vi "Dashboard Main.vi"() -> ()   [LabVIEW 2015]
uses:
  <vilib>/Utility/miscctls.llb/LVRowAndColumnTypeDef.ctl
  <vilib>/event_ctls.llb/eventvkey.ctl
  <vilib>/Rock Robotics/WPI/Dashboard/WPI_DashboardLogging Global.vi
  <vilib>/Rock Robotics/Network Tables/NT Read Numeric Array.vi
  <vilib>/Rock Robotics/Network Tables/NT Write Boolean.vi
  <vilib>/Utility/config.llb/Write Key (String).vi
  <vilib>/Utility/config.llb/Write Key (I32).vi
  <vilib>/Utility/config.llb/NI_LVConfig.lvlib
panel:
  in  "TCP":refnum<k5>
  in  "Rec Mode":enum32{"Stop", "Record", "Playback"}(radio)
  in  "Vision":u16(ring) items=["Camera Off", "USB Camera SW", "USB Camera HW", "IP Camera"]
  out "Camera IP":string
  out "Image Message":string="Timeout in Camera Communications"
  in  "Dashboard Tab":T1(tab)
  in  "Select Auto":string(combo)
  out "NT Connection":bool
  in  "Camera Settings":T2={"Frame Rate"=30, "Compression"=30, "Size"=1} {"Frame Rate" scale=1.0..30.0; "Size" items=["640x480", "320x240", "160x120"]}
  out "MotorChart R":cluster{"Numeric":dbl, "Numeric":dbl}(graph)
  out "MotorChart L":T3(graph)
  out "MotorSliders R":cluster{"MotorSlide1":dbl, "MotorSlide2":dbl} {"MotorSlide2" scale=-1.0..1.0 scale format="%#_2e"; "MotorSlide1" scale=-1.0..1.0 scale format="%#_2e"}
  out "MotorSliders L":T4 {"MotorSlide4 2" scale=0.0..14.0 scale format="%#_2e"; "MotorSlide2" scale=-1.0..1.0 scale format="%#_2e"; "MotorSlide1" scale=-1.0..1.0 scale format="%#_2e"}
  out "Gyro":dbl(knob) scale=0.0..360.0
  out "JS1 Z":dbl(slide) scale=-1.0..1.0 scale format="%#_2e"
  out "JS1 Graph":cluster{"X":dbl, "Y":dbl}[](graph)
  out "JS1 Buttons":T5
  out "JS2 Z":dbl(slide) scale=-1.0..1.0 scale format="%#_2e"
  out "JS2 Graph":cluster{"X":dbl, "Y":dbl}[](graph)
  out "JS2 Buttons":T5
  out "Mode":T6(ring)=enum."Auto Disabled"
  in  "DB Camera Config":bool
  out "fps":dbl format="%#.1g"
  out "Mbps":dbl format="%#.1g"
  out "Mbps LED":bool
  in  "Camera Switch":bool
  in  "Defenses":T7(ring)
  in  "Position":T8(ring)
  in  "DB/String 9":string
  in  "DB/String 8":string
  in  "DB/String 7":string
  in  "DB/String 6":string
  in  "DB/String 5":string
  in  "DB/String 4":string
  in  "DB/String 3":string
  in  "DB/String 2":string
  in  "DB/String 1":string
  in  "DB/String 0":string
  in  "DB/Slider 0":dbl(slide) scale=0.0..5.0
  in  "DB/Slider 1":dbl(slide) scale=0.0..5.0
  in  "DB/Slider 2":dbl(slide) scale=0.0..5.0
  in  "DB/Slider 3":dbl(slide) scale=0.0..5.0
  out "DB/LED 3":bool
  out "DB/LED 2":bool
  out "DB/LED 1":bool
  out "DB/LED 0":bool
  in  "DB/Button 3":bool
  in  "DB/Button 2":bool
  in  "DB/Button 1":bool
  in  "DB/Button 0":bool caption="New Name"
  in  "Test Slider":dbl(slide) scale=0.0..100.0 scale format="%#_3g"
  in  "On/Off":bool caption="Solenoid"
  in  "Test Name":u16(ring) items=["Select the test to run..."]
  in  "Test Tree":string(tree)
  in  "Motor":cluster{"Value":dbl, "Enable":bool} {"Value" scale=-1.0..1.0 scale format="%#_3g"}
  out "Progress":T9 {"Test Progress" scale=0.0..100.0}
  in  "Rev/Fwd":cluster{"Forward":bool, "Reverse":bool}
  in  "Test Ring":u16(ring) items=["Monochrome", "Color"]
  out "Cmd Status":string
  in  "Execute Command":bool
  in  "Command Params":string[][](table)
  in  "Command Selection":i32(listbox)
  in  "CheckList":i32(listbox)
  out "Tree":string(tree)
  out "Camera Image":T10(plugin-control)
  # "Left"
  # "Front"
  # "Right"
  # "Battery"
  # "This tab is a great place for autonomous settings and robot-specific values.\nPlace controls and indicators inside this tab and match name to\nDashboard Variables on robot. You can also delete this comment."
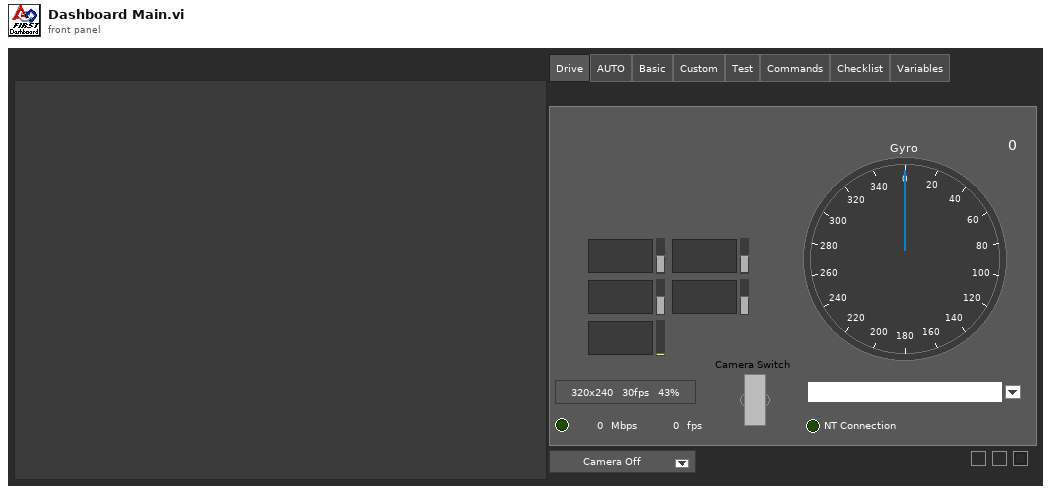
[diagram p1: front panel]
types:
  T1 = enum32{"Drive", "AUTO", "Basic", "Custom", "Test", "Commands", "Checklist", "Variables"}
  T2 = cluster{"Frame Rate":i32, "Compression":i32, "Size":u16}
  T3 = cluster{"Numeric":dbl, "Numeric":dbl, "Battery V":dbl}
  T4 = cluster{"MotorSlide1":dbl, "MotorSlide2":dbl, "MotorSlide4 2":dbl}
  T5 = cluster{bool, bool, bool, bool, bool, bool, bool, bool, bool, bool, bool, bool}
  T6 = enum8{"Tele-Op Disabled", "Tele-Op Enabled", "Auto Disabled", "Auto Enabled", "Test Disabled", "Test Enabled", "Disconnected", "No Code", "E-Stop"}
  T7 = enum16{"Sally Port", "Portcullis", "Drawbridge", "Moat", "Rock Wall", "Cheval De Frise", "Ramparts", "Low Bar", "Rocky Terrain"}
  T8 = enum16{"Position 5", "Position 4", "Position 3", "Position 2", "Position 1"}
  T9 = cluster{"Test Progress":u8, "Test Progress Text":string}
  T10 = typedef "IMAQ Image.ctl" = refnum<image>
  T11 = cluster{"IDs":cluster{"RPC field ID":u16, "Unique ID":u16}, "String":string}
  T12 = enum32{"Drive", "Basic", "Custom", "Test", "Checklist", "Variables"}
  T13 = typedef "Image Type" = u32
  T14 = cluster{"Error Strings":string, "Disable Counts":cluster{u16, u16}, "Rail Faults":cluster{u16, u16, u16}, "Robot IP":string, "DB Mode":u8, "Event Info":cluster{"Name":string, "Type":u8, "Number":u16, "Replay":u8}, "Camera Addr":string}
  T15 = cluster{"Storage":cluster{"Disk Free":u64, "RAM Block":u32, "RAM free":u32}, "CPU Utilization":cluster{"CPU % ISR":sgl, "CPU % Time Crit":sgl, "CPU % Timed Str":sgl, "CPU % High":sgl, "CPU % Above":sgl, "CPU % Normal":sgl, "CPU % Low":sgl}, "CAN":cluster{"% Bus Utilization":sgl, "Bus Off Cnt":u32, "TX_FIFO Full Cnt":u32, "Receive Error Cnt":u8, "Transmit Error Cnt":u8}, "HID":cluster{"HID Outputs":u32, "Rumble Low":u16, "Rumble High":u16}[]}
  T16 = cluster{"Status bits":cluster{"Test Mode":bool, "Autonomous":bool, "Enabled":bool, "Code Start":bool, "Brownout":bool, "Reserved 2":bool, "Reserved 3":bool, "E-Stop":bool}, "Code Trace":cluster{"Disabled":bool, "TeleOp":bool, "Auto":bool, "Test":bool}, "Controller Type":enum16{"unknown", "cRIO", "roboRio"}, "Code?":enum16{"unknown", "noCode", "code"}, "Battery V":dbl}
  T17 = cluster{"Control Bits":cluster{"TestMode":bool, "Autonomous":bool, "Enabled":bool, "FMS Present":bool, bool, bool, bool, "E-Stop":bool}, "Team Station ":u8, "Countdown":sgl, "Joystick Values":cluster{"Axes":dbl[], "Buttons":bool[], "POVs":i16[]}[]}
  T18 = cluster{"Axes":dbl[], "Buttons":bool[], "POVs":i16[]}[]
  T19 = cluster{"Axes":dbl[], "Buttons":bool[], "POVs":i16[]}
  T20 = cluster{"Buttons[0]":bool, "Buttons[1]":bool, "Buttons[2]":bool, "Buttons[3]":bool, "Buttons[4]":bool, "Buttons[5]":bool, "Buttons[6]":bool, "Buttons[7]":bool, "Buttons[8]":bool, "Buttons[9]":bool, "Buttons[10]":bool, "Buttons[11]":bool}
  T21 = typedef "NI_LVConfig.lvlib/Config Data RefNum.ctl" = refnum<k1>
  T22 = cluster{"Operation":enum16{"Update", "Clear"}, "Color Box":u32}[]
  T23 = typedef "eventvkey.ctl" = enum16{"ASCII", "Enter", "Return", "Shift", "Ctrl", "Alt", "Cmd", "Opt", "Caps", "NumLock", "Clear", "Break", "Up", "Down", "Left", "Right", "Insert", "Delete", "Home", "End", "PageUp", "PageDown", "Escape", "Help", "Pause", "ScrollLock", "F1", "F2", "F3", "F4", "F5", "F6", "F7", "F8", "F9", "F10", "F11", "F12", "F13", "F14", "F15", "F16", "F17", "F18", "F19", "F20", "F21", "F22", "F23", "F24", "Play", "VolumeUp", "VolumeDown", "Mute", "Two Byte Char"}
  T24 = cluster{"Image Size":bool, "Image Type":bool, "Pixel Value":bool, "ROI Information":bool, "Zoom Factor":bool}
  T25 = enum8{"Enabled", "Disabled", "Disabled and Grayed Out"}
  T26 = cluster{"Operation":enum16{"Update", "Clear"}, "Color Box":u32}
  T27 = typedef "LVRowAndColumnTypeDef.ctl" = cluster{"Row":i32, "Column":i32}
  T28 = cluster{"Shift":bool, "Ctrl":bool, "Alt":bool, "Cmd":bool, "Opt":bool}
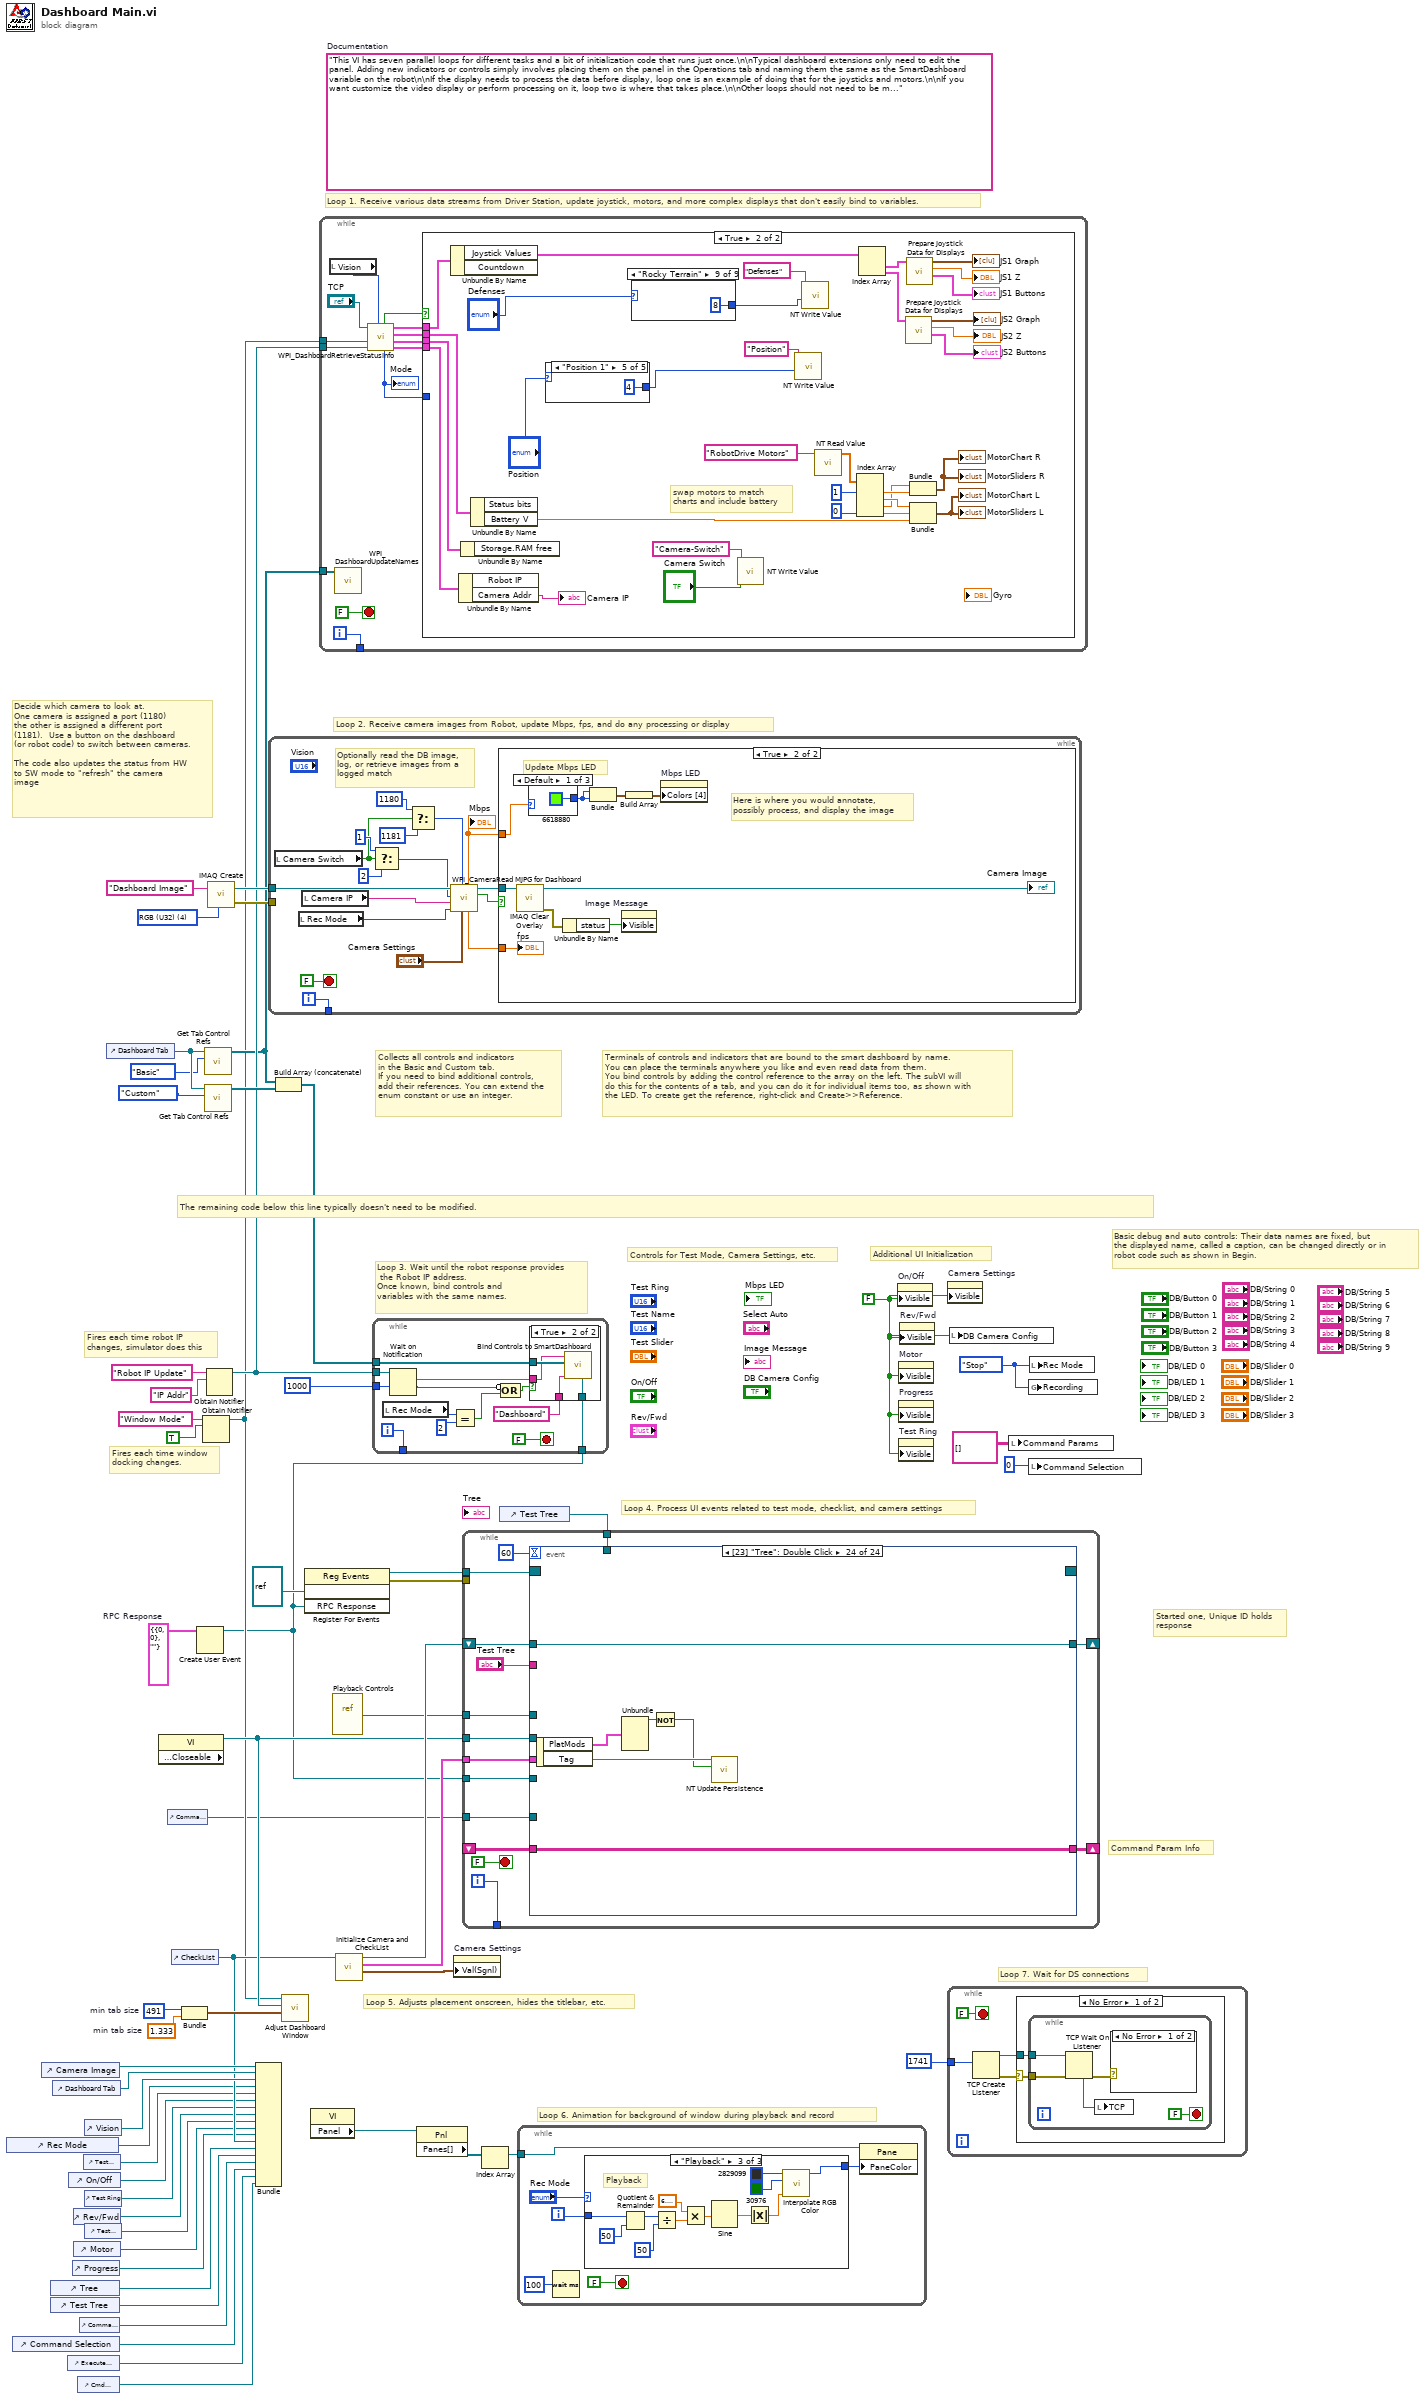
[diagram p0: block diagram]
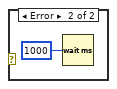
[diagram p2: hidden frame]
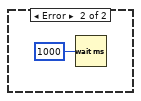
[diagram p3: hidden frame]
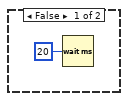
[diagram p4: hidden frame]
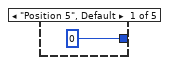
[diagram p5: hidden frame]
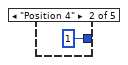
[diagram p6: hidden frame]
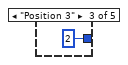
[diagram p7: hidden frame]
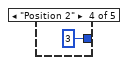
[diagram p8: hidden frame]
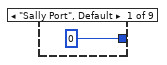
[diagram p9: hidden frame]
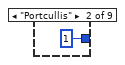
[diagram p10: hidden frame]
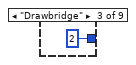
[diagram p11: hidden frame]
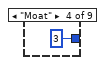
[diagram p12: hidden frame]
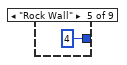
[diagram p13: hidden frame]
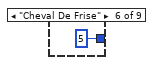
[diagram p14: hidden frame]
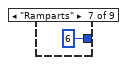
[diagram p15: hidden frame]
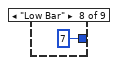
[diagram p16: hidden frame]
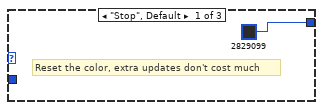
[diagram p17: hidden frame]
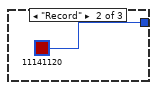
[diagram p18: hidden frame]
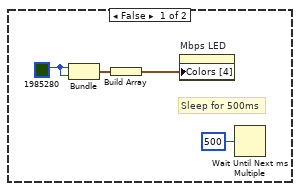
[diagram p20: hidden frame]
diagram:
  w7 = T11 {"IDs"={"RPC field ID"=0, "Unique ID"=0}, "String"=""}  # RPC Response
  w30 = 491  # min tab size
  w29 = 1.333  # min tab size
  w38 = enum32{"Stop", "Record", "Playback"}."Stop" ("Rec Mode")
  w14 = FALSE ("Visible")
  (unwired) "This VI has seven parallel loops for different tasks and a bit of initialization code that runs just once.\n\nTypical dashboard extensions only need to edit the panel. Adding new indicators or controls simply involves placing them on the panel in the Operations tab and naming them the same as the SmartDashboard variable on the robot\n\nIf the display needs to process the data before display, loop one is an example of doing that for the joysticks and motors.\n\nIf you want customize the video display or perform processing on it, loop two is where that takes place.\n\nOther loops should not need to be modified. They are pretty standard, and document the task they perform."  # Documentation
  w58 = T13 4 items=["Grayscale (U8)", "Grayscale (I16)", "Grayscale (SGL)", "Complex (CSG)", "RGB (U32)", "HSL (U32)", "RGB (U64)"] ("Image Type")
  # "Decide which camera to look at.\nOne camera is assigned a port (1180)\nthe other is assigned a different port\n(1181).  Use a button on the dashboard\n(or robot code) to switch between cameras.\n\nThe code also updates the status from HW\nto SW mode to \"refresh\" the camera\nimage"
  # "Command Param Info"
  # "Started one, Unique ID holds\nresponse"
  # "Loop 7. Wait for DS connections"
  # "Basic debug and auto controls: Their data names are fixed, but\nthe displayed name, called a caption, can be changed directly or in\nrobot code such as shown in Begin."
  # "Controls for Test Mode, Camera Settings, etc."
  # "Additional UI Initialization"
  # "Loop 6. Animation for background of window during playback and record"
  # "Fires each time robot IP\nchanges, simulator does this"
  # "Fires each time window\ndocking changes."
  # "Collects all controls and indicators\nin the Basic and Custom tab.\nIf you need to bind additional controls,\nadd their references. You can extend the\nenum constant or use an integer."
  # "The remaining code below this line typically doesn't need to be modified."
  # "Loop 4. Process UI events related to test mode, checklist, and camera settings"
  # "Terminals of controls and indicators that are bound to the smart dashboard by name.\nYou can place the terminals anywhere you like and even read data from them.\nYou bind controls by adding the control reference to the array on the left. The subVI will\ndo this for the contents of a tab, and you can do it for individual items too, as shown with\nthe LED. To create get the reference, right-click and Create>>Reference."
  # "Loop 3. Wait until the robot response provides\n the Robot IP address.\nOnce known, bind controls and\nvariables with the same names."
  # "Loop 5. Adjusts placement onscreen, hides the titlebar, etc."
  # "Loop 1. Receive various data streams from Driver Station, update joystick, motors, and more complex displays that don't easily bind to variables."
  # "Loop 2. Receive camera images from Robot, update Mbps, fps, and do any processing or display"
  n1 = control-ref of="Rec Mode"() -> (w20:refnum<vi>)
  n2 = control-ref of="Command Selection"() -> (w6:refnum<vi>)
  n3 = control-ref of="Camera Image"() -> (w33:refnum<vi>)
  n4 = control-ref of="Tree"() -> (w24:refnum<vi>)
  n5 = control-ref of="Test Tree"() -> (w23:refnum<vi>)
  n6 = control-ref of="Dashboard Tab"() -> (w32:refnum<vi>)
  n7 = control-ref of="Execute Command"() -> (w8:refnum<vi>)
  n8 = control-ref of="On/Off"() -> (w18:refnum<vi>)
  n9 = control-ref of="Progress"() -> (w15:refnum<vi>)
  n10 = control-ref of="Rev/Fwd"() -> (w16:refnum<vi>)
  n11 = control-ref of="Motor"() -> (w21:refnum<vi>)
  n12 = control-ref of="Cmd Status"() -> (w2:refnum<vi>)
  n13 = control-ref of="Command Params"() -> (w9:refnum<vi>)
  n14 = control-ref of="Test Slider"() -> (w19:refnum<vi>)
  n15 = control-ref of="Vision"() -> (w31:refnum<vi>)
  n16 = control-ref of="Test Ring"() -> (w17:refnum<vi>)
  n17 = control-ref of="Test Name"() -> (w22:refnum<vi>)
  n18 = control-ref of="Dashboard Tab"() -> (w36:refnum<vi>)
  n19 = property class="VI" props=["Front Panel.Closeable"]() -> (reference out=w37:refnum<vi>)  [unwired: 2 in, 2 out]
  n20 = control-ref of="Command Params"() -> (w1:refnum<vi>)
  n21 = control-ref of="CheckList"() -> (w25:refnum<vi>)
  n22 = Bundle("min tab size"=w30, "min tab size"=w29) -> (w28:cluster{"min tab size":i32, "min tab size":dbl})  [unwired: 1 in]
  n23 = Create User Event(user event datatype=w7) -> (user event=w3:refnum<user-event>)  [unwired: 1 in, 1 out]
  n24 = Obtain Notifier(name (unnamed)="Window Mode", notification data type=TRUE) -> (notifier out=w11:refnum<notifier>)  [unwired: 2 in, 2 out]
  n25 = call <vilib>:"Get Tab Control Refs.vi"("Page Index"=T12."Basic" ("Dashboard Tab"), "TabControl in"=w36) -> ("ControlsOnPage"=w12:refnum<vi>[])  [unwired: 9 in]
  n26 = call <vilib>:"Get Tab Control Refs.vi"("Page Index"=T12."Custom" ("Dashboard Tab"), "TabControl in"=w36) -> ("ControlsOnPage"=w35:refnum<vi>[])  [unwired: 9 in]
  n27 = Obtain Notifier(name (unnamed)="Robot IP Update", notification data type="IP Addr" ("name (unnamed)")) -> (notifier out=w13:refnum<notifier>)  [unwired: 2 in, 2 out]
  n28 = call "IMAQ Create"("Image Name"="Dashboard Image", "Image Type"=w58) -> ("New Image"=w56:T10, "error out"=w55:errorcluster)  [unwired: 2 in, 1 out]
  n29 = Bundle("Camera Image"=w33, "Dashboard Tab"=w32, "Vision"=w31, "Rec Mode"=w20, "Test Slider"=w19, "On/Off"=w18, "Test Ring"=w17, "Rev/Fwd"=w16, "Test Name"=w22, "Motor"=w21, "Progress"=w15, "CheckList"=w25, "Tree"=w24, "Test Tree"=w23, "Command Params"=w9, "Command Selection"=w6, "Execute Command"=w8, "Cmd Status"=w2) -> ()  [unwired: 1 in, 1 out]
  n30 = while {
    tunnel: w56 -> [w73]
    tunnel: w55 -> [_]
    tunnel: [w74] -> _
    i -> [w74]
    stop <- FALSE stop-if-true
    # "Optionally read the DB image,\nlog, or retrieve images from a\nlogged match"
    n31 = local read "Camera Switch"() -> (w60:bool)
    n32 = local read "Rec Mode"() -> (w68:enum32{"Stop", "Record", "Playback"})
    n33 = local read "Camera IP"() -> (w67:string)
    n34 = Select(t=1, s=w60, f=2) -> (s? t:f=w63:i32)
    n35 = Select(t=1180, s=w60, f=1181) -> (s? t:f=w59:i32)
    n36 = call <vilib>:"WPI_CameraRead MJPG for Dashboard.vi"("Camera Settings"="Camera Settings", "Camera Port"=w59, "Rec Mode"=w68, "Camera IP"=w67, "Camera Mode"=w63, "Refnum in"=w73) -> ("Active"=w71:bool, "Refnum out"=w72:T10, "FPS"=w70:dbl, "Bandwidth (Mbps)"=w66:dbl)  [unwired: 2 in]
    "Mbps" <- w66
    n37 = case shown="True" w71 {
      tunnel: w72 -> [_ w83]
      tunnel: w66 -> [_ w82]
      tunnel: w70 -> [_ w80]
      frame False {
        w76 = u32 1985280 ("Color Box")
        # "Sleep for 500ms"
        n38 = Bundle("Color Box"=w76, "Color Box"=w76) -> (w78:cluster{"Color Box":u32, "Color Box":u32})  [unwired: 1 out]
        n39 = Build Array(w78) -> (w77:cluster{"Color Box":u32, "Color Box":u32}[])
        n40 = property on="Mbps LED" class="Bool (strict)"("Colors [4]"=w77) -> ()  [unwired: 2 in, 2 out]
        n41 = Wait Until Next ms Multiple(millisecond multiple=u32 500) -> ()  [unwired: 1 out]
      }
      frame True {
        # "Here is where you would annotate,\npossibly process, and display the image"
        # "Update Mbps LED"
        n42 = call "IMAQ Clear Overlay"("Image"=w83) -> ("error out"=w87:errorcluster, "Image Out"=→"Camera Image":T10)  [unwired: 2 in, 7 out]
        n43 = case shown="Default" w82 {
          tunnel: [u32 6618880 ("Color Box") u32 16776722 ("Color Box") u32 16716800 ("Color Box")] -> w84
          frame Default {
          }
          frame 4, 5 {
          }
          frame 6.. {
          }
        }
        n44 = Unbundle By Name(w87) -> ("status"=w88:bool)
        n45 = Bundle("Color Box"=w84, "Color Box"=w84) -> (w86:cluster{"Color Box":u32, "Color Box":u32})  [unwired: 1 out]
        n46 = property on="Image Message" class="Str"("Visible"=w88) -> ()  [unwired: 2 in, 2 out]
        n47 = Build Array(w86) -> (w85:cluster{"Color Box":u32, "Color Box":u32}[])
        n48 = property on="Mbps LED" class="Bool (strict)"("Colors [4]"=w85) -> ()  [unwired: 2 in, 2 out]
        "fps" <- w80
      }
    }
  }
  n49 = Build Array (concatenate)(w12, w35) -> (w34:refnum<vi>[])
  n50 = call "Adjust Dashboard Window.vi"("Size Constraints"=w28, "VI"=w37, "WIn Mode"=w11) -> ()  [unwired: 9 in]
  n51 = register-events(refnum<vi> refnum, w3) -> (reference out=w42:refnum<event-registration>, error out=w41:errorcluster)  [unwired: 2 in]
  n52 = property class="VI"() -> ("Panel"=w45:refnum<vi>)  [unwired: 2 in, 2 out]
  n53 = while {
    tunnel: [w103] -> _
    tunnel: w13 -> [w97]
    tunnel: w12 -> [w96]
    tunnel: w11 -> [w92]
    i -> [w103]
    stop <- FALSE stop-if-true
    n54 = local read "Vision"() -> (w94:u16)
    n55 = call <vilib>:"WPI_DashboardUpdateNames.vi"("Controls on Tab"=w96) -> ()  [unwired: 11 in]
    n56 = call <vilib>:"WPI_DashboardRetrieveStatusInfo.vi"("Vision"=w94, "Binding Refnum"=w97, "Window Mode Notifier"=w92, "TCP Cnx"="TCP") -> ("Power and Errors"=w98:T14, "Robot Metrics"=w101:T15, "Status Info"=w102:T16, "Control Info"=w99:T17, "Robot Mode"=w95:T6, "Process?"=w100:bool)  [unwired: 2 in]
    "Mode" <- w95
    n57 = case shown="True" w100 {
      tunnel: w102 -> [_ w138]
      tunnel: w101 -> [_ w137]
      tunnel: w99 -> [_ w136]
      tunnel: w98 -> [_ w135]
      tunnel: w95 -> [_ _]
      frame False {
        n58 = Wait (ms)(milliseconds to wait=u32 20) -> ()  [unwired: 1 out]
      }
      frame True {
        # "swap motors to match\ncharts and include battery"
        n59 = Unbundle By Name(w136) -> ("Joystick Values"=w125:T18)  [unwired: 1 out]
        n60 = Unbundle By Name(w135) -> ("Camera Addr"=→"Camera IP":string)  [unwired: 1 out]
        n61 = Unbundle By Name(w137) -> ()  [unwired: 1 out]
        n62 = Unbundle By Name(w138) -> ("Battery V"=w126:dbl)  [unwired: 1 out]
        n63 = case shown="\"Position 1\"" "Position" {
          tunnel: [0 1 2 3 4] -> w106
          frame "Position 5", Default {
          }
          frame "Position 4" {
          }
          frame "Position 3" {
          }
          frame "Position 2" {
          }
          frame "Position 1" {
          }
        }
        n64 = case shown="\"Rocky Terrain\"" "Defenses" {
          tunnel: [0 1 2 3 4 5 6 7 8] -> w108
          frame "Sally Port", Default {
          }
          frame "Portcullis" {
          }
          frame "Drawbridge" {
          }
          frame "Moat" {
          }
          frame "Rock Wall" {
          }
          frame "Cheval De Frise" {
          }
          frame "Ramparts" {
          }
          frame "Low Bar" {
          }
          frame "Rocky Terrain" {
          }
        }
        n65 = call-poly <vilib>:"NT Write Value.vi"("Boolean"="Camera Switch", "Name"="Camera-Switch") -> ()  [unwired: 9 in, 1 out]
        n66 = call-poly <vilib>:"NT Write Value.vi"("Numeric"=w106, "Name"="Position") -> ()  [unwired: 9 in, 1 out]
        n67 = call-poly <vilib>:"NT Write Value.vi"("Numeric"=w108, "Name"="Defenses") -> ()  [unwired: 9 in, 1 out]
        n68 = call-poly <vilib>:"NT Read Value.vi"("Name"="RobotDrive Motors") -> ("Numeric Array"=w114:dbl[])  [unwired: 9 in, 1 out]
        n69 = Index Array(array=w114, index #1=1, index #4=0) -> (element #1=w130:dbl, element #2=w131:dbl, element #3=w129:dbl, element #4=w134:dbl)  [unwired: 2 in]
        n70 = Index Array(array=w125) -> (element #1=w124:T19, element #2=w119:T19)  [unwired: 2 in]
        n71 = call "Prepare Joystick Data for Displays.vi"("Joystick Values"=w119) -> ("Buttons"=→"JS2 Buttons":T20, "Z Axis"=→"JS2 Z":dbl, "Cartesian Data"=→"JS2 Graph":cluster{"X axis":dbl, "X axis":dbl}[])  [unwired: 8 in]
        n72 = call "Prepare Joystick Data for Displays.vi"("Joystick Values"=w124) -> ("Buttons"=→"JS1 Buttons":T20, "Z Axis"=→"JS1 Z":dbl, "Cartesian Data"=→"JS1 Graph":cluster{"X axis":dbl, "X axis":dbl}[])  [unwired: 8 in]
        n73 = Bundle("Numeric"=w129, "Numeric"=w130) -> (→"MotorChart R" →"MotorSliders R":cluster{"Numeric":dbl, "Numeric":dbl})  [unwired: 1 in]
        n74 = Bundle("Numeric"=w131, "Numeric"=w134, "Battery V"=w126) -> (→"MotorChart L" →"MotorSliders L":T3)  [unwired: 1 in]
      }
    }
  }
  n75 = vi-ref "Playback Controls.vi"() -> (w43:refnum<vi>)
  n76 = call "Initialize Camera and CheckList.vi"("ListBox in"=w25) -> ("Cluster"=w49:cluster{"value":i32, "value":i32, "index":i32}, "Array"=w50:cluster{string[]}[], "File Refnum"=w48:T21)  [unwired: 8 in]
  n77 = while {
    tunnel: w34 -> [w165]
    tunnel: w13 -> [w163]
    tunnel: [w161] -> _
    tunnel: u32 1000 ("milliseconds to wait") -> [w160]
    tunnel: w3 -> [w153]
    i -> [w161]
    stop <- FALSE stop-if-true
    n78 = local read "Rec Mode"() -> (w156:enum32{"Stop", "Record", "Playback"})
    n79 = Wait on Notification(notifier=w163, timeout in ms (-1)=w160) -> (notification=w162:string, timed out?=w158:bool)  [unwired: 2 in, 2 out]
    n80 = Equal?(x=w156, y=u16 2 ("Rec Mode")) -> (x = y?=w157:bool)
    n81 = Compound Arithmetic op=OR(invert w158, w157) -> (w159:bool)
    n82 = case shown="True" w159 {
      tunnel: w165 -> [_ w169]
      tunnel: w162 -> [_ w168]
      tunnel: "Dashboard" -> [_ w167]
      tunnel: w153 -> [_ w166]
      frame False {
      }
      frame True {
        n83 = call <vilib>:"Bind Controls to SmartDashboard.vi"("RPC ref"=w166, "Client Name"=w167, "Bound Control Refs"=w169, "Server IP Address"=w168) -> ()  [unwired: 8 in]
      }
    }
  }
  n84 = property class="Pnl"(reference=w45) -> ("Panes[]"=w46:refnum<vi>[])  [unwired: 1 in, 2 out]
  n85 = property on="Camera Settings" class="Clust (strict)"("Val(Sgnl)"=w49) -> ()  [unwired: 2 in, 2 out]
  n86 = Index Array(array=w46) -> (element=w44:refnum<vi>)  [unwired: 1 in]
  n87 = control-ref of="Test Tree"() -> (w47:refnum<vi>)
  n88 = while {
    tunnel: w50 -> [w181]
    shift-right: [w180] -> _
    shift-left: w48 -> [w179]
    tunnel: [w178] -> _
    tunnel: w47 -> [w177]
    tunnel: w43 -> [w176]
    tunnel: w42 -> [w175]
    tunnel: w41 -> [_]
    tunnel: w37 -> [w174]
    tunnel: w3 -> [w173]
    tunnel: w1 -> [w172]
    shift-right: [w171] -> _
    shift-left: _ -> [w170]
    i -> [w178]
    stop <- FALSE stop-if-true
    n89 = event shown="[23] \"Tree\": Double Click" {
      selector: w175 -> [_ _ _ _ _ _ _ _ _ _ _ _ _ _ _ _ _ _ _ _ _ _ _ _]
      dyn-events: [_ _ _ _ _ _ _ _ _ _ _ _ _ _ _ _ _ _ w490 _ _ _ _ _] -> _
      timeout: u32 60 ("milliseconds to wait") -> [_ _ _ _ _ _ _ _ _ _ _ _ _ _ _ _ _ _ _ _ _ _ _ _]
      tunnel: w177 -> [w194 _ _ _ _ _ _ _ _ _ _ _ _ _ _ _ _ _ _ _ _ _ _ _]
      tunnel: "Test Tree" -> [_ _ _ _ _ _ _ _ _ _ _ _ _ w453 w462 w465 w470 w479 _ _ _ _ _ _]
      tunnel: w181 -> [_ w232 _ _ _ _ _ _ _ _ _ w415 w446 _ _ _ _ _ _ _ _ _ _ _]
      tunnel: [w191 w231 w335 w341 w351 w355 w361 w373 w381 w387 w400 w414 w439 w452 w460 w464 w469 w478 w492 w508 w510 w518 w529 w534] -> w180
      tunnel: w179 -> [w191 w231 w335 w341 w351 w355 w361 w373 w381 w387 w400 w413 w439 w452 w460 w464 w469 w478 w492 w508 w510 w518 w529 w534]
      tunnel: w176 -> [_ _ _ _ _ _ _ _ _ _ _ _ _ _ _ _ _ _ w493 _ w513 _ _ _]
      tunnel: w174 -> [_ _ _ _ _ _ _ _ _ _ _ _ _ _ _ _ _ _ w488 _ _ _ _ _]
      tunnel: w173 -> [_ _ _ _ _ _ _ _ _ _ _ _ _ _ _ _ _ _ w484 _ _ _ _ _]
      tunnel: w172 -> [w186 _ _ _ _ _ w359 _ _ _ _ _ _ _ _ _ _ _ _ _ _ _ _ _]
      tunnel: [w185 w230 w334 w340 w350 w356 w357 w367 w378 w386 w399 w412 w438 w451 w459 w463 w468 w477 w483 w506 w509 w514 w522 w535] -> w171
      tunnel: w170 -> [w185 w230 w334 w340 w350 w356 w357 _ _ w386 w399 w412 w438 w451 w459 w463 w468 w477 w483 w506 w509 w514 w522 w535]
      event Timeout {
        n90 = event-data() -> ()  [unwired: 1 in, 1 out]
        n91 = local read "Mode"() -> (w188:T6)
        n92 = call <vilib>:"NT Read String.vi"("Name"="/TestMode/TestName") -> ("String"=w197:string)  [unwired: 9 in, 1 out]
        n93 = case shown="\"Test\"" "Dashboard Tab" {
          tunnel: w194 -> [_ w208 _ _]
          tunnel: "/TestMode/Automatic/" ("Name Pattern") -> [_ w207 _ _]
          tunnel: T22 [{"Operation"=enum."Clear", "Color Box"=14013909}, {"Operation"=enum."Clear", "Color Box"=14013909}, {"Operation"=enum."Clear", "Color Box"=14013909}, {"Operation"=enum."Clear", "Color Box"=14013909}, {"Operation"=enum."Update", "Color Box"=14013909}, {"Operation"=enum."Update", "Color Box"=16777215}, {"Operation"=enum."Clear", "Color Box"=14013909}, {"Operation"=enum."Clear", "Color Box"=14013909}, {"Operation"=enum."Clear", "Color Box"=14013909}] -> [_ w200 _ w217]
          tunnel: w188 -> [_ w199 _ w216]
          tunnel: u32[] [15790320, 15790320, 15790320, 15790320, 16777215, 16777215, 15790320, 15790320, 15790320] -> [_ _ _ w222]
          tunnel: w186 -> [_ _ _ w210]
          frame "Custom", Default {
          }
          frame "Test" {
            w206 = -2 ("Active Item:Row Number")
            n94 = Index Array(array=w200, index=w199) -> (element=w201:T26)
            n95 = Unbundle(w201) -> ("Operation"=w202:enum16{"Update", "Clear"}, "Color Box"=w203:u32)
            n96 = call <vilib>:"NT Read and Format Entries as Tree.vi"("Operation"=w202, "Name Pattern"=w207, "Tree Refnum"=w208) -> ()  [unwired: 7 in, 2 out]
            n97 = property on="Test Tree" class="Tree (strict)"("Active Item Row Number"=w206, "ActiveColNum"=w206, "CellBG"=w203, "Active Item Row Number"=-1 ("Active Item:Row Number"), "CellBG"=u32 5789784 ("Color Box")) -> ()  [unwired: 2 in, 2 out]
          }
          frame "Variables" {
            n98 = control-ref of="Tree"() -> (w209:refnum<vi>)
            n99 = call <vilib>:"NT Read and Format Entries as Tree.vi"("Tree Refnum"=w209) -> ()  [unwired: 9 in, 2 out]
          }
          frame "Commands" {
            w218 = u32 5789784 ("Color Box")
            w219 = T27 {"Row"=-1, "Column"=-2} ("Active Cell:Active Cell")
            w221 = T27 {"Row"=-2, "Column"=-2} ("Active Cell:Active Cell")
            n100 = Index Array(array=w222, index=w216) -> (element=w220:u32)
            n101 = Index Array(array=w217, index=w216) -> (element=w215:T26)
            n102 = Unbundle(w215) -> ("Operation"=w214:enum16{"Update", "Clear"})  [unwired: 1 out]
            n103 = local read "Command Selection"() -> (w213:i32)
            n104 = property on="Command Selection" class="MCListbox (strict)"("ActiveCell"=w221, "CellBG"=w220, "ActiveCell"=w219, "CellBG"=w218) -> ()  [unwired: 2 in, 2 out]
            n105 = call <vilib>:"WPI_DashboardUpdate RPC Info.vi"("Operation"=w214) -> ("update"=w212:bool, "commands"=w211:string[][])  [unwired: 9 in]
            n106 = property on="Command Selection" class="MCListbox (strict)"("ItemNames"=w211) -> ()  [unwired: 2 in, 2 out]
            n107 = property on="Command Params" class="Tbl (strict)"("Active Cell"=w221, "Cell BG Color"=w220, "Active Cell"=w219, "Cell BG Color"=w218) -> ()  [unwired: 2 in, 2 out]
            n108 = call <vilib>:"WPI_DashboardUpdate Command Params.vi"("Update"=w212, "NewVal"=w213, "Commands"=w211, "Param Tbl"=w210) -> ()  [unwired: 7 in, 1 out]
          }
        }
        n109 = case shown="\"\"" w197 {
          tunnel: "/TestMode/TestProgress" ("Name") -> [w224 _]
          tunnel: "/TestMode/TestProgressText" ("Name") -> [w223 _]
          frame Default {
            n110 = call <vilib>:"NT Read Number.vi"("Name"=w224) -> ("Numeric"=w225:dbl)  [unwired: 9 in, 1 out]
            n111 = call <vilib>:"NT Read String.vi"("Name"=w223) -> ("String"=w226:string)  [unwired: 9 in, 1 out]
            n112 = Bundle("Numeric"=w225, "String"=w226) -> (→"Progress":cluster{"Numeric":dbl, "String":string})  [unwired: 1 in]
          }
          frame "" {
            n113 = property on="Progress" class="Clust (strict)"("Visible"=FALSE) -> ()  [unwired: 2 in, 2 out]
            n114 = local write "Test Name"(u16 0) -> ()
          }
        }
        n115 = call <vilib>:"Connextion Info.vi"() -> ("Connected"=→"NT Connection":bool)  [unwired: 10 in, 1 out]
      }
      event "Test Tree": Value Change {
        # "Show appropriate\ncontrols"
        n116 = event-data() -> ("CtlRef"=w235:refnum<vi>, "NewVal"=w233:string)  [unwired: 1 in]
        n117 = call <vilib>:"WPI_UtilitiesGetTreeIOName.vi"("NewVal"=w233, "TreeControl in"=w235) -> ("I/O Name"=w236:string)  [unwired: 9 in]
        n118 = case shown="\"Analog Out\", \"Motor\", \"PWM\"" w236 {
          selector: w236 -> [_ w243 _ w265 w274 _]
          tunnel: w233 -> [_ _ w262 w264 _ w281]
          tunnel: w232 -> [_ _ _ _ _ w280]
          frame Default {
            w238 = FALSE ("Visible")
            w237 = FALSE ("Visible")
            n119 = property on="Motor" class="Clust (strict)"("Visible"=w237) -> ()  [unwired: 2 in, 2 out]
            n120 = property on="Test Ring" class="Ring (strict)"("Visible"=w237) -> ()  [unwired: 2 in, 2 out]
            n121 = property on="Rev/Fwd" class="Clust (strict)"("Visible"=w238) -> ()  [unwired: 2 in, 2 out]
            n122 = property on="On/Off" class="Bool (strict)"("Visible"=w238) -> ()  [unwired: 2 in, 2 out]
            n123 = property on="Test Slider" class="Slide (strict)"("Visible"=w238) -> ()  [unwired: 2 in, 2 out]
          }
          frame "Analog Out", "Motor", "PWM" {
            w244 = FALSE ("Visible")
            n124 = case shown="\"Analog Out\"" w243 {
              tunnel: [1.0 ("Value") -1.0 ("Value") 0.0 ("Value")] -> w242
              tunnel: [255.0 ("Value") 1.0 ("Value") 5.0 ("Value")] -> w241
              tunnel: [128.0 ("Value") 0.0 ("Value") 0.0 ("Value")] -> w240
              tunnel: [64.0 ("Value") 0.5 ("Value") 1.0 ("Value")] -> w239
              frame "PWM" {
              }
              frame "Motor", Default {
              }
              frame "Analog Out" {
              }
            }
            n125 = property on="Motor" class="Clust (strict)"("Visible"=TRUE) -> ()  [unwired: 2 in, 2 out]
            n126 = property on="Value" class="Slide (strict)"("Value"=w240, "Scale.Minimum"=w242, "Scale.Maximum"=w241, "Scale.Increment"=w239) -> ()  [unwired: 2 in, 2 out]
            n127 = property on="On/Off" class="Bool (strict)"("Visible"=w244) -> ()  [unwired: 2 in, 2 out]
            n128 = property on="Test Slider" class="Slide (strict)"("Visible"=w244) -> ()  [unwired: 2 in, 2 out]
            n129 = property on="Test Ring" class="Ring (strict)"("Visible"=w244) -> ()  [unwired: 2 in, 2 out]
            n130 = property on="Rev/Fwd" class="Clust (strict)"("Visible"=w244) -> ()  [unwired: 2 in, 2 out]
          }
          frame "Servo" {
            w260 = FALSE ("Visible")
            n131 = call <vilib>:"NT Read Number.vi"("Name"=w262) -> ("Numeric"=w261:dbl)  [unwired: 9 in, 1 out]
            n132 = property on="Test Slider" class="Slide (strict)"("Visible"=TRUE, "Scale.Maximum"=170.0 ("Scale.Range:Maximum")) -> ()  [unwired: 2 in, 2 out]
            n133 = local write "Test Slider"(w261) -> ()
            n134 = property on="Motor" class="Clust (strict)"("Visible"=w260) -> ()  [unwired: 2 in, 2 out]
            n135 = property on="Rev/Fwd" class="Clust (strict)"("Visible"=w260) -> ()  [unwired: 2 in, 2 out]
            n136 = property on="On/Off" class="Bool (strict)"("Visible"=w260) -> ()  [unwired: 2 in, 2 out]
            n137 = property on="Test Ring" class="Ring (strict)"("Visible"=w260) -> ()  [unwired: 2 in, 2 out]
          }
          frame "Relay", "Solenoid" {
            w263 = FALSE ("Visible")
            n138 = property on="Motor" class="Clust (strict)"("Visible"=w263) -> ()  [unwired: 2 in, 2 out]
            n139 = property on="Test Slider" class="Slide (strict)"("Visible"=w263) -> ()  [unwired: 2 in, 2 out]
            n140 = Search and Replace String(input string=w264, search string="/Value  **", replace string="/Direction") -> (result string=w270:string)  [unwired: 5 in, 3 out]
            n141 = property on="Test Ring" class="Ring (strict)"("Visible"=w263) -> ()  [unwired: 2 in, 2 out]
            n142 = call <vilib>:"NT Read String.vi"("Name"=w270) -> ("String"=w268:string)  [unwired: 9 in, 1 out]
            n143 = Equal?(x="Both directions", y=w268) -> (x = y?=w266:bool)
            n144 = Not(x=w266) -> (.not. x?=w267:bool)
            n145 = property on="Rev/Fwd" class="Clust (strict)"("Visible"=w266) -> ()  [unwired: 2 in, 2 out]
            n146 = property on="On/Off" class="Bool (strict)"("Visible"=w267, "Caption.Text"=w265) -> ()  [unwired: 2 in, 2 out]
          }
          frame "Compressor", "Digital Out" {
            w273 = FALSE ("Visible")
            # "Get direction and finish"
            n147 = property on="Motor" class="Clust (strict)"("Visible"=w273) -> ()  [unwired: 2 in, 2 out]
            n148 = property on="Test Slider" class="Slide (strict)"("Visible"=w273) -> ()  [unwired: 2 in, 2 out]
            n149 = property on="Test Ring" class="Ring (strict)"("Visible"=w273) -> ()  [unwired: 2 in, 2 out]
            n150 = property on="On/Off" class="Bool (strict)"("Visible"=TRUE, "Caption.Text"=w274) -> ()  [unwired: 2 in, 2 out]
            n151 = property on="Rev/Fwd" class="Clust (strict)"("Visible"=FALSE) -> ()  [unwired: 2 in, 2 out]
          }
          frame "Camera" {
            n152 = call <vilib>:"Get Last Path Segment.vi"("String in"=w281) -> ("String out"=w282:string)  [unwired: 10 in]
            n153 = property on="On/Off" class="Bool (strict)"("Visible"=FALSE) -> ()  [unwired: 2 in, 2 out]
            n154 = property on="Motor" class="Clust (strict)"("Visible"=FALSE) -> ()  [unwired: 2 in, 2 out]
            n155 = property on="Rev/Fwd" class="Clust (strict)"("Visible"=FALSE) -> ()  [unwired: 2 in, 2 out]
            n156 = case shown="\"White Balance  **\"" w282 {
              tunnel: w281 -> [w288 w297 w306 w315 w324 _ w330]
              tunnel: w280 -> [w286 w294 w303 w312 w321 _ _]
              frame "Size  **" {
                n157 = Index Array(array=w286) -> (element=w285:cluster{string[]})  [unwired: 1 in]
                n158 = call <vilib>:"NT Read String.vi"("Name"=w288) -> ("String"=w287:string)  [unwired: 9 in, 1 out]
                n159 = Unbundle(w285) -> (w283:string[])
                n160 = Match First String(2:w283, 3:w287) -> (0:w284:i32)  [unwired: 1 out]
                n161 = property on="Test Ring" class="Ring (strict)"("Value"=w284, "Strings []"=w283) -> ()  [unwired: 2 in, 2 out]
                n162 = property on="Test Ring" class="Ring (strict)"("Visible"=TRUE) -> ()  [unwired: 2 in, 2 out]
                n163 = property on="Test Slider" class="Slide (strict)"("Visible"=FALSE) -> ()  [unwired: 2 in, 2 out]
              }
              frame "White Balance  **" {
                n164 = Index Array(array=w294, index=1) -> (element=w295:cluster{string[]})
                n165 = call <vilib>:"NT Read String.vi"("Name"=w297) -> ("String"=w296:string)  [unwired: 9 in, 1 out]
                n166 = Unbundle(w295) -> (w292:string[])
                n167 = Match First String(2:w292, 3:w296) -> (0:w291:i32)  [unwired: 1 out]
                n168 = property on="Test Ring" class="Ring (strict)"("Value"=w291, "Strings []"=w292) -> ()  [unwired: 2 in, 2 out]
                n169 = property on="Test Ring" class="Ring (strict)"("Visible"=TRUE) -> ()  [unwired: 2 in, 2 out]
                n170 = property on="Test Slider" class="Slide (strict)"("Visible"=FALSE) -> ()  [unwired: 2 in, 2 out]
              }
              frame "Exposure  **" {
                n171 = Index Array(array=w303, index=2) -> (element=w304:cluster{string[]})
                n172 = call <vilib>:"NT Read String.vi"("Name"=w306) -> ("String"=w305:string)  [unwired: 9 in, 1 out]
                n173 = Unbundle(w304) -> (w300:string[])
                n174 = Match First String(2:w300, 3:w305) -> (0:w301:i32)  [unwired: 1 out]
                n175 = property on="Test Ring" class="Ring (strict)"("Value"=w301, "Strings []"=w300) -> ()  [unwired: 2 in, 2 out]
                n176 = property on="Test Ring" class="Ring (strict)"("Visible"=TRUE) -> ()  [unwired: 2 in, 2 out]
                n177 = property on="Test Slider" class="Slide (strict)"("Visible"=FALSE) -> ()  [unwired: 2 in, 2 out]
              }
              frame "Exposure Priority  **" {
                n178 = Index Array(array=w312, index=3) -> (element=w313:cluster{string[]})
                n179 = call <vilib>:"NT Read String.vi"("Name"=w315) -> ("String"=w314:string)  [unwired: 9 in, 1 out]
                n180 = Unbundle(w313) -> (w309:string[])
                n181 = Match First String(2:w309, 3:w314) -> (0:w310:i32)  [unwired: 1 out]
                n182 = property on="Test Ring" class="Ring (strict)"("Value"=w310, "Strings []"=w309) -> ()  [unwired: 2 in, 2 out]
                n183 = property on="Test Ring" class="Ring (strict)"("Visible"=TRUE) -> ()  [unwired: 2 in, 2 out]
                n184 = property on="Test Slider" class="Slide (strict)"("Visible"=FALSE) -> ()  [unwired: 2 in, 2 out]
              }
              frame "Color Enable  **" {
                n185 = Index Array(array=w321, index=4) -> (element=w322:cluster{string[]})
                n186 = call <vilib>:"NT Read String.vi"("Name"=w324) -> ("String"=w323:string)  [unwired: 9 in, 1 out]
                n187 = Unbundle(w322) -> (w318:string[])
                n188 = Match First String(2:w318, 3:w323) -> (0:w319:i32)  [unwired: 1 out]
                n189 = property on="Test Ring" class="Ring (strict)"("Value"=w319, "Strings []"=w318) -> ()  [unwired: 2 in, 2 out]
                n190 = property on="Test Ring" class="Ring (strict)"("Visible"=TRUE) -> ()  [unwired: 2 in, 2 out]
                n191 = property on="Test Slider" class="Slide (strict)"("Visible"=FALSE) -> ()  [unwired: 2 in, 2 out]
              }
              frame Default {
                n192 = property on="Test Ring" class="Ring (strict)"("Visible"=FALSE) -> ()  [unwired: 2 in, 2 out]
                n193 = property on="Test Slider" class="Slide (strict)"("Visible"=FALSE) -> ()  [unwired: 2 in, 2 out]
              }
              frame "Brightness  **", "Color Level  **", "Compression  **", "FPS  **", "Sharpness  **" {
                n194 = call <vilib>:"NT Read Number.vi"("Name"=w330) -> ("Numeric"=w329:dbl)  [unwired: 9 in, 1 out]
                n195 = local write "Test Slider"(w329) -> ()
                n196 = property on="Test Slider" class="Slide (strict)"("Visible"=TRUE, "Scale.Maximum"=100.0 ("Scale.Range:Maximum")) -> ()  [unwired: 2 in, 2 out]
                n197 = property on="Test Ring" class="Ring (strict)"("Visible"=FALSE) -> ()  [unwired: 2 in, 2 out]
              }
            }
          }
        }
        n198 = property on="Progress" class="Clust (strict)"("Visible"=FALSE) -> ()  [unwired: 2 in, 2 out]
      }
      event "Test Name": Mouse Enter {
        # "Populate the ring with the list of tests"
        n199 = event-data() -> ()  [unwired: 1 in, 1 out]
        n200 = call <vilib>:"NT Read String Array.vi"("Name"="/TestMode/TestList") -> ("String Array"=w339:string[])  [unwired: 9 in, 1 out]
        n201 = Build Array (concatenate)("Select the test to run...", w339) -> (w338:string[])
        n202 = property on="Test Name" class="Ring (strict)"("Strings []"=w338) -> ()  [unwired: 2 in, 2 out]
      }
      event "Test Name": Value Change {
        w342 = FALSE ("Visible")
        # "Tell the robot the test name to run"
        n203 = event-data() -> ("NewVal"=w346:u16)  [unwired: 1 in]
        n204 = property on="Test Name" class="Ring (strict)"() -> ("Strings []"=w347:string[])  [unwired: 2 in, 2 out]
        n205 = local write "Progress"(T9 {"Test Progress"=0, "Test Progress Text"=""} ("Progress")) -> ()
        n206 = Index Array(array=w347, index=w346) -> (element=w345:string)
        n207 = call <vilib>:"NT Write String.vi"("String"=w345, "Name"="/TestMode/TestName") -> ()  [unwired: 9 in, 1 out]
        n208 = property on="Progress" class="Clust (strict)"("Visible"=TRUE) -> ()  [unwired: 2 in, 2 out]
        n209 = property on="Motor" class="Clust (strict)"("Visible"=w342) -> ()  [unwired: 2 in, 2 out]
        n210 = property on="Test Slider" class="Slide (strict)"("Visible"=w342) -> ()  [unwired: 2 in, 2 out]
        n211 = property on="On/Off" class="Bool (strict)"("Visible"=w342) -> ()  [unwired: 2 in, 2 out]
        n212 = property on="Rev/Fwd" class="Clust (strict)"("Visible"=w342) -> ()  [unwired: 2 in, 2 out]
        n213 = property on="Test Ring" class="Ring (strict)"("Visible"=w342) -> ()  [unwired: 2 in, 2 out]
      }
      event "Select Auto": Mouse Enter {
        # "Populate the combo box with the list of autonomous options"
        n214 = event-data() -> ()  [unwired: 1 in, 1 out]
        n215 = call <vilib>:"NT Read String Array.vi"("Name"="Auto List") -> ("String Array"=w349:string[])  [unwired: 9 in, 1 out]
        n216 = property on="Select Auto" class="CmbBox"("Strings[]"=w349) -> ()  [unwired: 2 in, 2 out]
      }
      event "Select Auto": Value Change {
        # "User modified the Auto Selection. Write to NT variable so robot knows."
        n217 = event-data() -> ("NewVal"=w353:string)  [unwired: 1 in]
        n218 = call <vilib>:"NT Write String.vi"("String"=w353, "Name"="Auto Selector") -> ()  [unwired: 9 in, 1 out]
      }
      event "Command Selection": Value Change {
        # "Get the params and show in table"
        n219 = event-data() -> ("NewVal"=w360:i32)  [unwired: 1 in]
        n220 = property on="Command Selection" class="MCListbox (strict)"() -> ("ItemNames"=w358:string[][])  [unwired: 2 in, 2 out]
        n221 = call <vilib>:"WPI_DashboardUpdate Command Params.vi"("NewVal"=w360, "Commands"=w358, "Param Tbl"=w359) -> ()  [unwired: 8 in, 1 out]
      }
      event "Execute Command": Value Change {
        # "Started one, Unique ID holds\nresponse"
        n222 = event-data() -> ()  [unwired: 1 in, 1 out]
        n223 = property on="Command Selection" class="MCListbox (strict)"() -> ("ItemNames"=w372:string[][])  [unwired: 2 in, 2 out]
        n224 = Index Array(array=w372, index (row)="Command Selection", index (col)=0) -> (element=w370:string)
        n225 = call <vilib>:"Invoke Commands.vi"("Command Params"="Command Params", "Function Name"=w370) -> ("Params"=w366:u8, "Started"=w365:bool)  [unwired: 7 in, 1 out]
        n226 = Array Subset(array="Command Params", length (row)=w366) -> (w367:string[][])  [unwired: 3 in]
        n227 = Select(t="Executing" ("Cmd Status"), s=w365, f="" ("Cmd Status")) -> (s? t:f=→"Cmd Status":string)
      }
      event "Command Selection": Double Click {
        n228 = event-data() -> ("Row"=w382:i32)  [unwired: 1 in]
        n229 = property on="Command Selection" class="MCListbox (strict)"() -> ("ItemNames"=w385:string[][])  [unwired: 2 in, 2 out]
        n230 = local read "Command Params"() -> (w380:string[][])
        n231 = Index Array(array=w385, index (row)=w382, index (col)=0) -> (element=w383:string)
        n232 = call <vilib>:"Invoke Commands.vi"("Command Params"=w380, "Function Name"=w383) -> ("Params"=w379:u8, "Started"=w374:bool)  [unwired: 7 in, 1 out]
        n233 = Array Subset(array=w380, length (row)=w379) -> (w378:string[][])  [unwired: 3 in]
        n234 = Select(t="Executing" ("Cmd Status"), s=w374, f="" ("Cmd Status")) -> (s? t:f=w375:string)
        n235 = local write "Cmd Status"(w375) -> ()
      }
      event "CheckList": Double Click {
        # "Shift clears all"
        # "Update symbols on the listbox"
        n236 = event-data() -> ("PlatMods.Shift"=w388:bool, "Row"=w390:i32)  [unwired: 1 in]
        n237 = case shown="True" w388 {
          tunnel: w390 -> [w394 _]
          tunnel: 1 -> [w393 _]
          frame False {
            n238 = property on="CheckList" class="LstBox (strict)"() -> ("Item Symbols"=w392:i32[])  [unwired: 2 in, 2 out]
            n239 = Replace Array Subset(array=w392, new element=w393, index=w394) -> (w391:i32[])
            n240 = property on="CheckList" class="LstBox (strict)"("Item Symbols"=w391) -> ()  [unwired: 2 in, 2 out]
          }
          frame True {
            w395 = 0 ("Top Row")
            n241 = property on="CheckList" class="LstBox (strict)"() -> ("Number of Rows"=w397:u32)  [unwired: 2 in, 2 out]
            n242 = Initialize Array(0, w397) -> (w396:i32[])
            n243 = property on="CheckList" class="LstBox (strict)"("Top Row"=w395, "Value"=w395, "Item Symbols"=w396) -> ()  [unwired: 2 in, 2 out]
          }
        }
      }
      event "CheckList": Key Down {
        # "Update symbols on the listbox\nLeft and right keys check and uncheck"
        n244 = event-data() -> ("VKey"=w402:T23)  [unwired: 1 in]
        n245 = case shown="\"Left\", \"Right\"" w402 {
          selector: w402 -> [w407 _]
          tunnel: eventvkey."Left" ("VKey") -> [w405 _]
          frame "Left", "Right" {
            n246 = Equal?(x=w405, y=w407) -> (x = y?=w406:bool)
            n247 = Select(t=0, s=w406, f=1) -> (s? t:f=w408:i32)
            n248 = property on="CheckList" class="LstBox (strict)"() -> ("Item Symbols"=w411:i32[])  [unwired: 2 in, 2 out]
            n249 = Replace Array Subset(array=w411, new element=w408, index="CheckList") -> (w410:i32[])
            n250 = property on="CheckList" class="LstBox (strict)"("Item Symbols"=w410) -> ()  [unwired: 2 in, 2 out]
          }
          frame Default {
          }
        }
      }
      event "DB Camera Config": Value Change {
        # "Show or hide the cluster of controls, store in ini file"
        n251 = event-data() -> ("NewVal"=w416:bool)  [unwired: 1 in]
        n252 = case shown="False" w416 {
          tunnel: w415 -> [w425 _]
          tunnel: [w418 w436] -> w414
          tunnel: w413 -> [w417 w436]
          frame False {
            w432 = "Camera"
            w435 = FALSE ("Visible")
            n253 = local read "Camera Settings"() -> (w424:T2)
            n254 = Index Array(array=w425) -> (element=w428:cluster{string[]})  [unwired: 1 in]
            n255 = Unbundle(w424) -> ("Frame Rate"=w423:i32, "Compression"=w422:i32, "Size"=w426:u16)
            n256 = Unbundle(w428) -> (w427:string[])
            n257 = Index Array(array=w427, index=w426) -> (element=w421:string)
            n258 = call-poly <vilib>:"Write Key.vi"("section"=w432, "value"=w421, "key"="Size", "refnum"=w417) -> ("refnum out"=w434:T21)  [unwired: 2 in, 5 out]
            n259 = call-poly <vilib>:"Write Key.vi"("section"=w432, "value"=w423, "key"="FrameRate", "refnum"=w434) -> ("refnum out"=w433:T21)  [unwired: 1 in, 6 out]
            n260 = property on="Camera Settings" class="Clust (strict)"("Visible"=w435) -> ()  [unwired: 2 in, 2 out]
            n261 = local write "DB Camera Config"(w435) -> ()
            n262 = call-poly <vilib>:"Write Key.vi"("section"=w432, "value"=w422, "key"="Compression", "refnum"=w433) -> ("refnum out"=w419:T21)  [unwired: 1 in, 6 out]
            n263 = call <vilib>:"Close Config Data.vi"("refnum"=w419) -> ("file path"=w420:path)  [unwired: 2 in, 8 out]
            n264 = call <vilib>:"Open Config Data.vi"("configuration file path"=w420) -> ("refnum"=w418:T21)  [unwired: 8 in, 2 out]
          }
          frame True {
            n265 = property on="Camera Settings" class="Clust (strict)"("Visible"=TRUE) -> ()  [unwired: 2 in, 2 out]
          }
        }
      }
      event "Camera Settings": Value Change {
        # "Update summary string when any elements of DB camera change"
        n266 = event-data() -> ("NewVal"=w450:T2)  [unwired: 1 in]
        n267 = Index Array(array=w446) -> (element=w445:cluster{string[]})  [unwired: 1 in]
        n268 = Unbundle(w450) -> ("Frame Rate"=w441:i32, "Compression"=w440:i32, "Size"=w443:u16)
        n269 = Unbundle(w445) -> (w444:string[])
        n270 = Index Array(array=w444, index=w443) -> (element=w442:string)
        n271 = Format Into String(format string="%s   %dfps   %d%%", w442, w441, w440) -> (resulting string=w447:string)  [unwired: 2 in, 1 out]
        n272 = Build Array(w447) -> (w448:string[])
        n273 = property on="DB Camera Config" class="Bool (strict)"("Strings [4]"=w448) -> ()  [unwired: 2 in, 2 out]
      }
      event "Motor.Enable": Value Change {
        # "When the test mode otor enable helper is set, update that\ntree row item's value"
        n274 = event-data() -> ("NewVal"=w457:bool)  [unwired: 1 in]
        n275 = Unbundle("Motor") -> ("Value"=w456:dbl)  [unwired: 1 out]
        n276 = Select(t=w456, s=w457, f=0.0) -> (s? t:f=w454:dbl)
        n277 = call <vilib>:"NT Write Number.vi"("Numeric"=w454, "Name"=w453) -> ()  [unwired: 9 in, 1 out]
      }
      event "Test Slider": Value Change {
        # "When the test mode slider helper is set, update that\ntree row item's value"
        n278 = event-data() -> ("NewVal"=w461:dbl)  [unwired: 1 in]
        n279 = call <vilib>:"NT Write Number.vi"("Numeric"=w461, "Name"=w462) -> ()  [unwired: 9 in, 1 out]
      }
      event "On/Off": Value Change {
        # "When the test mode on/off helper value is set, update that\ntree row item's value"
        n280 = event-data() -> ("NewVal"=w467:bool)  [unwired: 1 in]
        n281 = Boolean To (0,1)(Boolean=w467) -> (0, 1=w466:i16)
        n282 = call <vilib>:"NT Write Number.vi"("Numeric"=w466, "Name"=w465) -> ()  [unwired: 9 in, 1 out]
      }
      event "Rev/Fwd": Value Change {
        # "When the test mode helper value for relays is set, update that\ntree row item's value"
        n283 = event-data() -> ("NewVal.Forward"=w476:bool, "NewVal.Reverse"=w475:bool)  [unwired: 1 in]
        n284 = Boolean To (0,1)(Boolean=w476) -> (0, 1=w472:i16)
        n285 = Boolean To (0,1)(Boolean=w475) -> (0, 1=w474:i16)
        n286 = Negate(x=w474) -> (-x=w473:i16)
        n287 = Add(x=w472, y=w473) -> (x+y=w471:i16)
        n288 = call <vilib>:"NT Write Number.vi"("Numeric"=w471, "Name"=w470) -> ()  [unwired: 9 in, 1 out]
      }
      event "Test Ring": Value Change {
        # "When a test mode helper value is selected from the ring,\nset the tree item's variable to the string value"
        n289 = event-data() -> ("NewVal"=w481:u16)  [unwired: 1 in]
        n290 = property on="Test Ring" class="Ring (strict)"() -> ("Strings []"=w482:string[])  [unwired: 2 in, 2 out]
        n291 = Index Array(array=w482, index=w481) -> (element=w480:string)
        n292 = call <vilib>:"NT Write String.vi"("String"=w480, "Name"=w479) -> ()  [unwired: 9 in, 1 out]
      }
      event "Rec Mode": Value Change {
        # "Update globals for recording mode and path to read log from.\nClear when logging and let NetworkTables set path for vision to\nuse."
        n293 = event-data() -> ("NewVal"=w494:enum32{"Stop", "Record", "Playback"})  [unwired: 1 in]
        n294 = global write "WPI_DashboardLogging Global.vi" "Logging Filename"(path "") -> ()
        n295 = global write "WPI_DashboardLogging Global.vi" "Recording"(w494) -> ()
        n296 = case shown="\"Playback\"" w494 {
          tunnel: w493 -> [_ w496 w505]
          tunnel: [_ _ w504] -> w490
          tunnel: [_ _ w503] -> _
          tunnel: w488 -> [_ _ w501]
          tunnel: cluster{i32, i32} {-250, 170} -> [_ _ w500]
          tunnel: [_ _ T24 {"Image Size"=TRUE, "Image Type"=TRUE, "Pixel Value"=TRUE, "ROI Information"=TRUE, "Zoom Factor"=FALSE} ("Image Information Shown:All Elements")] -> w486
          tunnel: [_ _ TRUE ("Zoom Factor")] -> w485
          tunnel: w484 -> [_ _ w497]
          frame Default {
          }
          frame "Stop", "Record" {
            # "Place Window too"
            n297 = invoke class="VI" method="FP.Close"(reference=w496) -> (reference out=w495:refnum<vi>)  [unwired: 2 in, 2 out]
            n298 = invoke class="VI" method="Abort VI"(reference=w495) -> ()  [unwired: 2 in, 3 out]
          }
          frame "Playback" {
            n299 = call "Open Playback Panel.vi"("Offset"=w500, "DB VI Ref"=w501, "Playback in"=w505) -> ("Playback out"=w502:refnum<vi>)  [unwired: 8 in]
            n300 = register-events(w502, w497) -> (reference out=w504:refnum<event-registration>, error out=w503:errorcluster)  [unwired: 2 in]
          }
        }
        n301 = property on="Camera Image" class="ImageControl"("Image Information Shown"=w486, "Image Information Visible"=w485) -> ()  [unwired: 2 in, 2 out]
        n302 = call <vilib>:"WPI_DashboardNT Log FieldName Cache.vi"("Operation"=enum16{"Lookup/Add", "Index", "Clear"}."Clear") -> ()  [unwired: 8 in, 3 out]
      }
      event Panel Close {
        w507 = enum32{"Stop", "Record", "Playback"}."Stop" ("Rec Mode")
        # "Playback window has been closed, abort"
        n303 = event-data() -> ()  [unwired: 1 in, 4 out]
        n304 = local write "Rec Mode"(w507) -> ()
        n305 = global write "WPI_DashboardLogging Global.vi" "Recording"(w507) -> ()
      }
      event Panel Close {
        # "Abort playback window and ourself"
        n306 = event-data() -> ()  [unwired: 1 in, 4 out]
        n307 = invoke class="VI" method="FP.Close"(reference=w513) -> (reference out=w512:refnum<vi>)  [unwired: 2 in, 2 out]
        n308 = invoke class="VI" method="Abort VI"(reference=w512) -> (error out=w511:errorcluster)  [unwired: 2 in, 2 out]
        n309 = invoke class="VI" method="Abort VI"(error in=w511) -> ()  [unwired: 2 in, 3 out]
      }
      event User Event {
        n310 = event-data() -> ("IDs"=w521:cluster{"RPC field ID":u16, "Unique ID":u16}, "String"=w520:string)  [unwired: 1 in]
        n311 = Bundle("IDs"=w521, "String"=w520) -> (w519:T11)  [unwired: 1 in]
        n312 = call <vilib>:"Retrieve RPC Response.vi"("RPC Response"=w519) -> ("Output"=w516:string[][])  [unwired: 10 in]
        n313 = Build Array (concatenate)(w514, w516) -> (w515:string[][])
        n314 = local write "Command Params"(w515) -> ()
        n315 = local write "Cmd Status"("" ("Cmd Status")) -> ()
      }
      event "Vision": Value Change {
        # "Enable/Disable Compression slider.\nHW USB is hard-coded into the camera"
        n316 = event-data() -> ("NewVal"=w528:u16)  [unwired: 1 in]
        n317 = Equal?(x=w528, y=u32 2 ("milliseconds to wait")) -> (x = y?=w526:bool)
        n318 = Select(t=T25."Disabled and Grayed Out" ("Disabled"), s=w526, f=T25."Enabled" ("Disabled")) -> (s? t:f=w523:T25)
        n319 = property on="Compression" class="Slide (strict)"("DisabledEnum"=w523) -> ()  [unwired: 2 in, 2 out]
      }
      event "Tree": Double Click {
        n320 = event-data() -> ("PlatMods"=w533:T28, "Tag"=w532:string)  [unwired: 1 in]
        n321 = Unbundle(w533) -> ("Shift"=w531:bool)  [unwired: 4 out]
        n322 = Not(x=w531) -> (.not. x?=w530:bool)
        n323 = call <vilib>:"NT Update Persistence.vi"("Persistence"=w530, "Name"=w532) -> ()  [unwired: 9 in, 1 out]
      }
    }
  }
  n324 = while {
    tunnel: w44 -> [w537]
    i -> [w540]
    stop <- FALSE stop-if-true
    n325 = Wait (ms)(milliseconds to wait=u32 100) -> ()  [unwired: 1 out]
    n326 = case shown="\"Playback\"" "Rec Mode" {
      tunnel: w540 -> [_ _ w555]
      tunnel: [u32 2829099 ("Base Color") u32 11141120 ("Target Color") w544] -> w536
      frame "Stop", Default {
        # "Reset the color, extra updates don't cost much"
      }
      frame "Record" {
      }
      frame "Playback" {
        # "Playback"
        n327 = Quotient & Remainder(x=w555, y=u32 50 ("milliseconds to wait")) -> (x-y*floor(x/y)=w551:u32)  [unwired: 1 out]
        n328 = Divide(x=w551, y=u32 50 ("milliseconds to wait")) -> (x/y=w548:dbl)
        n329 = Multiply(x=6.283185307179586, y=w548) -> (x*y=w553:dbl)
        n330 = Sine(x=w553) -> (sin(x)=w552:dbl)
        n331 = Absolute Value(x=w552) -> (abs(x)=w545:dbl)
        n332 = call "Interpolate RGB Color.vi"("Proportion"=w545, "Target Color"=u32 30976, "Base Color"=u32 2829099) -> ("Result Color"=w544:u32)  [unwired: 8 in]
      }
    }
    n333 = property class="Pane"(reference=w537, "PaneColor"=w536) -> ()  [unwired: 1 in, 2 out]
  }
  n334 = property on="On/Off" class="Bool (strict)"("Visible"=w14) -> ()  [unwired: 2 in, 2 out]
  n335 = property on="Motor" class="Clust (strict)"("Visible"=w14) -> ()  [unwired: 2 in, 2 out]
  n336 = property on="Progress" class="Clust (strict)"("Visible"=w14) -> ()  [unwired: 2 in, 2 out]
  n337 = property on="Test Ring" class="Ring (strict)"("Visible"=w14) -> ()  [unwired: 2 in, 2 out]
  n338 = property on="Rev/Fwd" class="Clust (strict)"("Visible"=w14) -> ()  [unwired: 2 in, 2 out]
  n339 = property on="Camera Settings" class="Clust (strict)"("Visible"=w14) -> ()  [unwired: 2 in, 2 out]
  n340 = while {
    tunnel: u16 1741 ("timeout ms (25000)") -> [w557]
    stop <- FALSE stop-if-true
    n341 = TCP Create Listener(10:w557) -> (0:w556:errorcluster, 3:w558:refnum<k5>)  [unwired: 4 in, 1 out]
    n342 = case shown="No Error" w556 {
      selector: w556 -> [w560 _]
      tunnel: w558 -> [w561 _]
      frame No Error {
        n343 = while {
          tunnel: w561 -> [w564]
          tunnel: w560 -> [w563]
          stop <- FALSE stop-if-true
          n344 = TCP Wait On Listener(8:w563, 11:w564) -> (0:w565:errorcluster, 4:w566:refnum<k5>)  [unwired: 2 in, 3 out]
          n345 = local write "TCP"(w566) -> ()
          n346 = case shown="No Error" w565 {
            frame No Error {
            }
            frame Error {
              n347 = Wait (ms)(milliseconds to wait=u32 1000) -> ()  [unwired: 1 out]
            }
          }
        }
      }
      frame Error {
        n348 = Wait (ms)(milliseconds to wait=u32 1000) -> ()  [unwired: 1 out]
      }
    }
  }
  n349 = local write "DB Camera Config"(w14) -> ()
  n350 = local write "Command Params"(string[][] [] ("Command Params")) -> ()
  n351 = global write "WPI_DashboardLogging Global.vi" "Recording"(w38) -> ()
  n352 = local write "Command Selection"(u16 0 ("milliseconds to wait")) -> ()
  n353 = local write "Rec Mode"(w38) -> ()
